vi "UpdateDisplayBuffer.vi"(8 "FilteredAndRectified":waveform(dbl)[](graph) caption="Filtered\nand\nRectified", 9 "dispSize":dbl=20.0 caption="Lower Cut-Off", 10 "MVC Data":cluster{"queue out":refnum<queue>, dbl, dbl}[](array[cluster]), 11 "Disp Data":cluster{"queue out":refnum<queue>, dbl, dbl}[](array[cluster])) -> (2 "Disp Data Out":cluster{"queue out":refnum<queue>, dbl, dbl}[](array[cluster]))   [LabVIEW 2016]
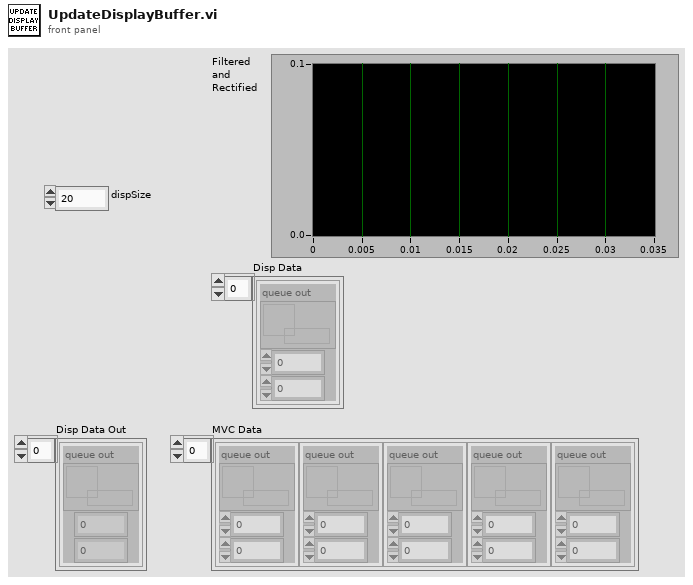
[diagram p1: front panel]
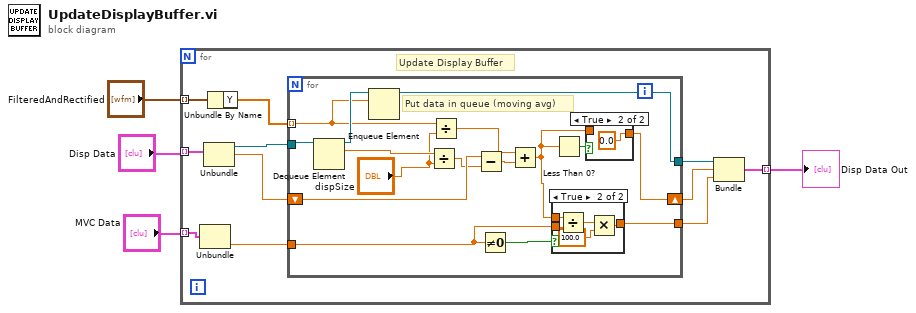
[diagram p0: block diagram]
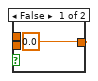
[diagram p3: hidden frame]
diagram:
  n1 = for {
    tunnel: "Disp Data" -> [w9] mode=indexing
    tunnel: "FilteredAndRectified" -> [w14] mode=indexing
    tunnel: [w10] -> w3 mode=indexing
    tunnel: "MVC Data" -> [w7] mode=indexing
    # "Update Display Buffer"
    n2 = Unbundle(w7) -> (w6:dbl)  [unwired: 2 out]
    n3 = Unbundle(w9) -> ("queue out"=w15:refnum<queue>, w8:dbl)  [unwired: 1 out]
    n4 = Unbundle By Name(w14) -> ("Y"=w13:dbl[])
    n5 = for {
      tunnel: w15 -> [w26]
      tunnel: w13 -> [w22] mode=indexing
      shift-right: [w17] -> w12
      shift-left: w8 -> [w30]
      tunnel: [w21] -> w11
      tunnel: w6 -> [w24]
      tunnel: [w20] -> w5
      # "Put data in queue (moving avg)"
      n6 = Dequeue Element(queue=w26) -> (queue out=w23:refnum<queue>, element=w31:dbl)  [unwired: 2 in, 2 out]
      n7 = Enqueue Element(queue=w23, element=w22) -> (queue out=w21:refnum<queue>)  [unwired: 2 in, 2 out]
      n8 = Divide(x=w31, y="dispSize") -> (x/y=w29:dbl)
      n9 = Divide(x=w22, y="dispSize") -> (x/y=w27:dbl)
      n10 = Subtract(x=w30, y=w29) -> (x-y=w28:dbl)
      n11 = Not Equal To 0?(x=w24) -> (x != 0?=w25:bool)
      n12 = Add(x=w27, y=w28) -> (x+y=w18:dbl)
      n13 = case shown="True" w25 {
        tunnel: w24 -> [_ w39]
        tunnel: [0.0 w37] -> w20
        tunnel: w18 -> [_ w38]
        frame False {
        }
        frame True {
          n14 = Divide(x=w38, y=w39) -> (x/y=w36:dbl)
          n15 = Multiply(x=w36, y=100.0) -> (x*y=w37:dbl)
        }
      }
      n16 = Less Than 0?(x=w18) -> (x < 0?=w19:bool)
      n17 = case shown="True" w19 {
        tunnel: [w32 0.0] -> w17
        tunnel: w18 -> [w32 _]
        frame False {
        }
        frame True {
        }
      }
    }
    n18 = Bundle("queue out"=w11, w12, w5) -> (w10:cluster{"queue out":refnum<queue>, dbl, dbl})  [unwired: 1 in]
  }
  "Disp Data Out" <- w3
